vi "tsapp_get_bus_statistics.vi"(7 "AIdxStat":i32(ring) items=["cbsBusLoad", "cbsPeakLoad", "cbsFpsStdData", "cbsAllStdData", "cbsFpsExtData", "cbsAllExtData", "cbsFpsStdRemote", "cbsAllStdRemote", "cbsFpsExtRemote", "cbsAllExtRemote", "cbsFpsErrorFrame", "cbsAllErrorFrame"], 8 "error in (no error)":errorcluster caption="错误输入（无错误）", 9 "AIdxChn":i32(ring) items=["CHN1", "CHN2", "CHN3", "CHN4", "CHN5", "CHN6", "CHN7", "CHN8", "CHN9", "CHN10", "CHN11", "CHN12", "CHN13", "CHN14", "CHN15", "CHN16", "CHN17", "CHN18", "CHN19", "CHN20", "CHN21", "CHN22", "CHN23", "CHN24", "CHN25", "CHN26", "CHN27", "CHN28", "CHN29", "CHN30", "CHN31", "CHN32"], 10 "ABusType":i32(ring) items=["APP_CAN", "APP_LIN"], 11 "路径输入":path) -> (0 "error out":errorcluster caption="错误输出", 1 "AStat":dbl, 2 "retuen":i32, 3 "路径输出":path)   [LabVIEW 2014]
doc: "Function Introduction :\nObtain bus statistics\nCall location :\ninput parameter :\nABusType: Application Channel Type\nAIdxChn: Channel index starts from 0\nAIdxStat: Bus Statistics Index\nAStat: retrieved status values\nReturn value :\n==0: Execution successful\nOther values: Query error code\n\nCbsBusLoad: Bus load, which may indicate the current load situation on the CAN bus (percentage of bandwidth occupied).\nCbsPeakLoad: Peak load, representing the highest load of the CAN bus during a certain period of time.\nCbsFpsStdData: The frame rate per second of standard data frames, which calculates the transmission rate of standard data frames (ID 11 bits).\nCbsAllStdData: The total number of standard data frames, representing the total number of standard data frames in the statistical process.\nCbsFpsExtData: The frame rate per second of the extended data frame, which calculates the transmission rate of the extended data frame (ID 29 bits).\nCbsAllExtData: The total number of extended data frames, representing the total number of extended data frames during the statistical process.\nCbsFpsStdRemote: The frame rate per second of standard remote frames, and the sending rate of standard remote frames.\nCbsAllStdRemote: The total number of standard remote frames, representing the total number of standard remote frames during the statistical process.\nCbsFpsExtRemote: Extend the frame rate of remote frames per second and calculate the sending rate of extended remote frames.\nCbsAllExtRemote: The total number of extended remote frames, representing the total number of extended remote frames during the statistical process.\nCbsFpsError Frame: The frame rate per second of error frames, which calculates the sending rate of error frames (CAN error frames).\nCbsAllError Frame: The total number of error frames, representing the total number of error frames in the statistical process."
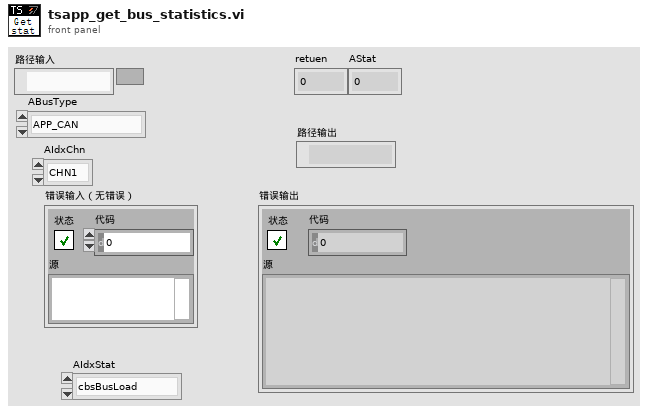
[diagram p1: front panel]
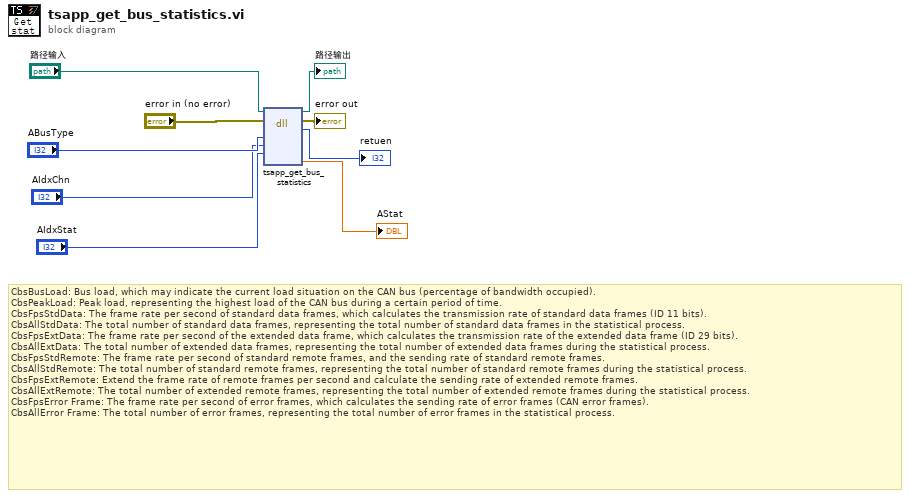
[diagram p0: block diagram]
diagram:
  # "CbsBusLoad: Bus load, which may indicate the current load situation on the CAN bus (percentage of bandwidth occupied).\nCbsPeakLoad: Peak load, representing the highest load of the CAN bus during a certain period of time.\nCbsFpsStdData: The frame rate per second of standard data frames, which calculates the transmission rate of standard data frames (ID 11 bits).\nCbsAllStdData: The total number of standard data frames, representing the total number of standard data frames in the statistical process.\nCbsFpsExtData: The frame rate per second of the extended data frame, which calculates the transmission rate of the extended data frame (ID 29 bits).\nCbsAllExtData: The total number of extended data frames, representing the total number of extended data frames during the statistical process.\nCbsFpsStdRemote: The frame rate per second of standard remote frames, and the sending rate of standard remote frames.\nCbsAllStdRemote: The total number of standard remote frames, representing the total number of standard remote frames during the statistical process.\nCbsFpsExtRemote: Extend the frame rate of remote frames per second and calculate the sending rate of extended remote frames.\nCbsAllExtRemote: The total number of extended remote frames, representing the total number of extended remote frames during the statistical process.\nCbsFpsError Frame: The frame rate per second of error frames, which calculates the sending rate of error frames (CAN error frames).\nCbsAllError Frame: The total number of error frames, representing the total number of error frames in the statistical process."
  n1 = dll-call lib="D:/Work/LabVIEW Code/TSMaster Labview SDK/LabVIEW/LabVIEW-TSMasterAPI_CLN/TSMasterAPI_LabVIEW-2024-08-02 09-14-06/Not_organized_vi/TSMaster.*" fn="tsapp_get_bus_statistics"(path in="路径输入", error in="error in (no error)", "ABusType"="ABusType", "AIdxChn"="AIdxChn", "AIdxStat"="AIdxStat") -> (path out=→"路径输出":path, error out=→"error out":errorcluster, "返回类型"=→"retuen":i32, "AStat"=→"AStat":dbl)  [unwired: 5 in]
